vi "VMI_move_1_delay.vi"(5 "Postion / mm":refnum<vi>, 6 "Target Offset / mm":dbl=-0.1, 7 "Stop":refnum<vi>, 8 "Error In":errorcluster, 9 "Target Position / mm":dbl, 10 "Repeat Velocity / mms-1":dbl=3.0, 11 "Delay Cluster":T1={"System no."=1, "Identification"="Physik Instrumente, C-843,21200023, V2.1.2.0", "Device ID out"=0, "Postion / mm"=[10.0], "SN out"="", "Movement Range"=[50.0], "Conn. Axes"=["1"], "Target Position / mm"=10.0, "Velocity / mm s^-1"=0.5, "Set-up"=TRUE, "Moving"=FALSE, "Step Size / mm "=0.15, "Stage Number"=0, "Polling Time /ms"=0, "Delay Scan?"=TRUE, "Accurate Scan"=FALSE, "CmdMovDelay"=FALSE, "CmdStopDelay"=FALSE, "Delay List"=[["Number", "Target / mm", "Relative Integration Time"]], "Scan Start /mm"=50.0, "Scan End / mm"=80.0}) -> (0 "error out":errorcluster)   [LabVIEW 2017]
uses:
  Type defs/PI_delay_settings_alt.ctl
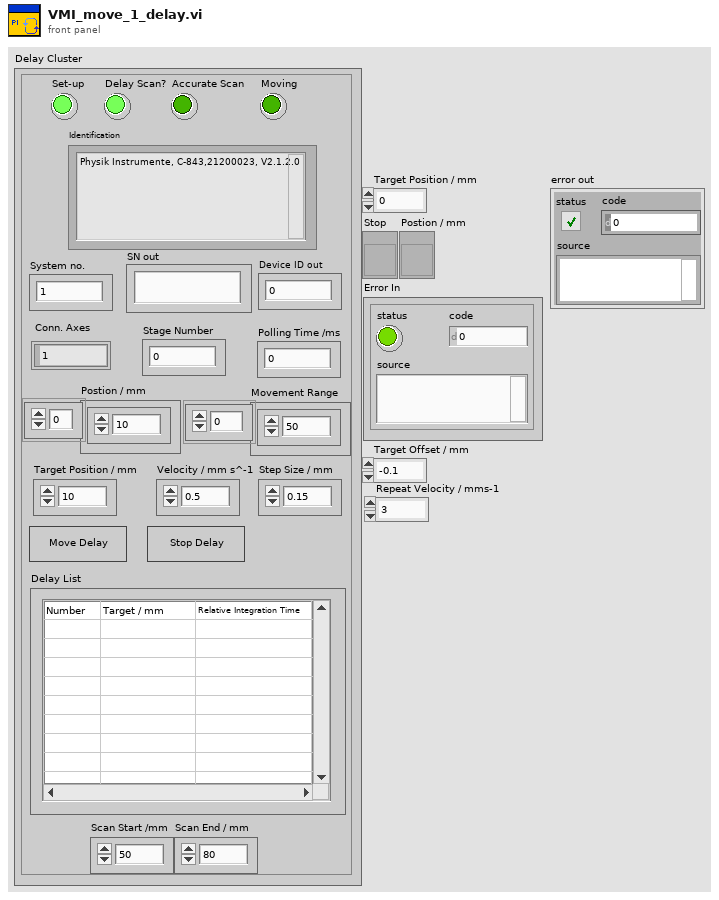
[diagram p1: front panel]
types:
  T1 = typedef "PI_delay_settings_alt.ctl" = cluster{"System no.":i32, "Identification":string, "Device ID out":i32, "Postion / mm":dbl[], "SN out":string, "Movement Range":dbl[], "Conn. Axes":string[], "Target Position / mm":dbl, "Velocity / mm s^-1":dbl, "Set-up":bool, "Moving":bool, "Step Size / mm ":dbl, "Stage Number":i32, "Polling Time /ms":i32, "Delay Scan?":bool, "Accurate Scan":bool, "CmdMovDelay":bool, "CmdStopDelay":bool, "Delay List":string[][], "Scan Start /mm":dbl, "Scan End / mm":dbl}
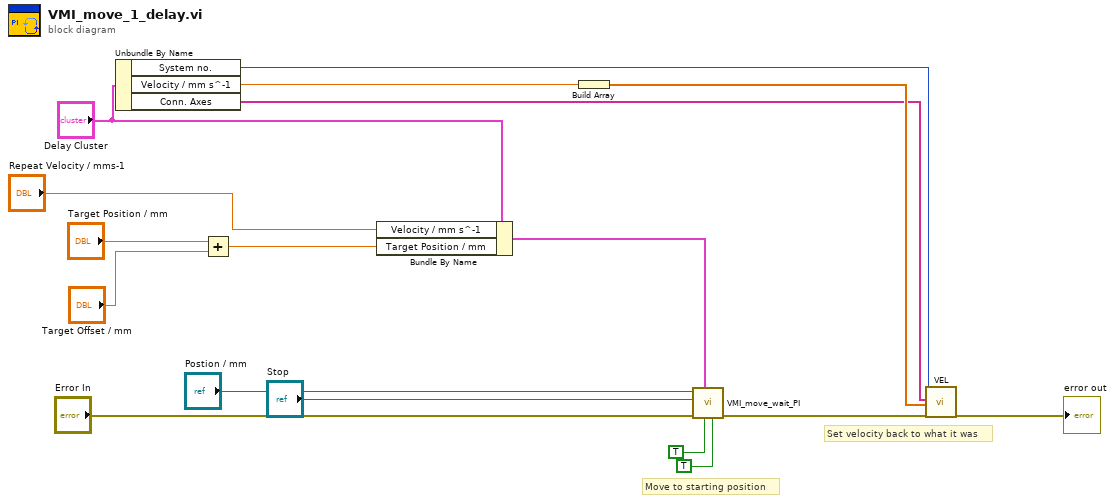
[diagram p0: block diagram]
diagram:
  # "Move to starting position"
  # "Set velocity back to what it was"
  n1 = Unbundle By Name("Delay Cluster") -> ("System no."=w4:i32, "Velocity / mm s^-1"=w6:dbl, "Conn. Axes"=w3:string[])
  n2 = Add(x="Target Position / mm", y="Target Offset / mm") -> (x+y=w10:dbl)
  n3 = Bundle By Name(cluster="Delay Cluster", "Velocity / mm s^-1"="Repeat Velocity / mms-1", "Target Position / mm"=w10) -> (w17:T1)
  n4 = Build Array(w6) -> (w5:dbl[])
  n5 = call "VMI_move_wait_PI.vi"("SetV?"=TRUE, "Move and Wait?"=TRUE, "Delay Cluster"=w17, "Error In"="Error In", "Stop ref"="Stop", "Postion / mm"="Postion / mm") -> ("error out"=w2:errorcluster)  [unwired: 5 in]
  n6 = call "VEL.vi"("System no."=w4, "Axes to set"=w3, "Velocity values"=w5, "error in"=w2) -> ("error out"=→"error out":errorcluster)  [unwired: 2 in, 13 out]
